vi "vPage_9222x1_CHx1.vi"() -> ()   [LabVIEW 2022 SP3]
uses:
  <vilib>/Utility/sysdir.llb/System Directory Type.ctl
  <vilib>/express/express analysis/Spectral/Block/exnSpectralBlock spectral measurements peak poly.vi
  <vilib>/express/express analysis/Spectral/Block/exnSpectralBlock spectral measurements peak DDT.vi
  <vilib>/express/express analysis/Spectral/XNode/ExpressSpectralMeasurementsBlockNode.xnode
panel:
  out "Buffer":i32
  in  "device name":tag="cDAQ8Mod1"
  in  "FFT":bool
  in  "¸ê®Æ§¨\nµù°O>":string
  out "DAQ Stoped":bool
  in  "Sample \nto Read":i32=200000
  in  "Sample\nRate":dbl=200000.0
  in  "Enable Saving":bool
  in  "Stop":bool
  out "C1-Save":bool
  out "C1-Trigger":bool
  out "C1-0":dynamicdata(graph)
  out "C1-1":dynamicdata(graph)
  # "關閉FFT\n可提高效率"
  # "當 Buffer 不為零時\n存檔&畫面會有延遲"
  # "本頁畫面顯示為 觸發後訊號"
  # "FFT Filter by useing High-pass with Lower Cut-Off (Hz)"
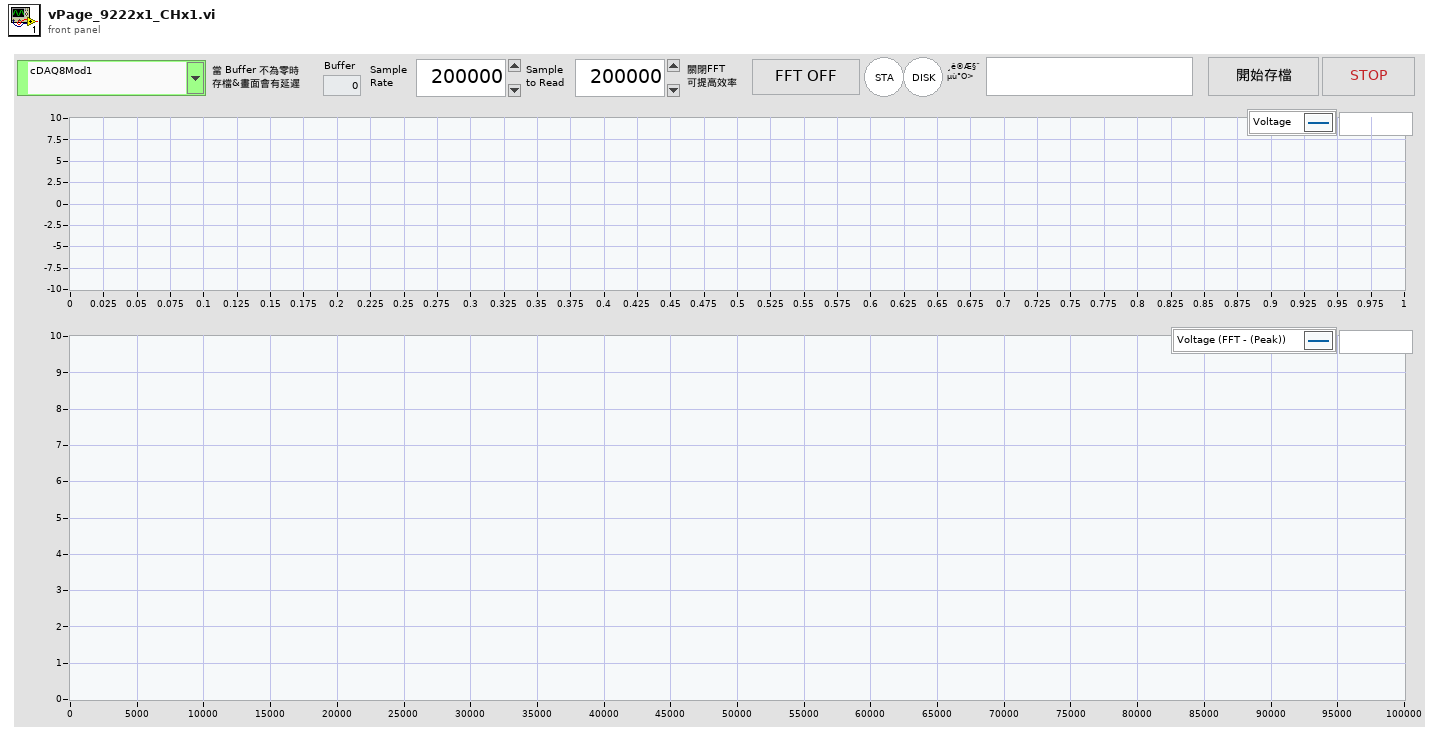
[diagram p1: front panel]
types:
  T1 = enum8{"Enabled", "Disabled", "Disabled and Grayed Out"}
  T2 = typedef "System Directory Type.ctl" = i32
  T3 = cluster{"task out":refnum<k21>, "data":dynamicdata}
  T4 = cluster{"averaging mode":u16, "weighting mode":u16, "number of averages":u32}
  T5 = cluster{"dB On (F)":bool, "unwrap phase (F)":bool, "convert to degree (F)":bool}
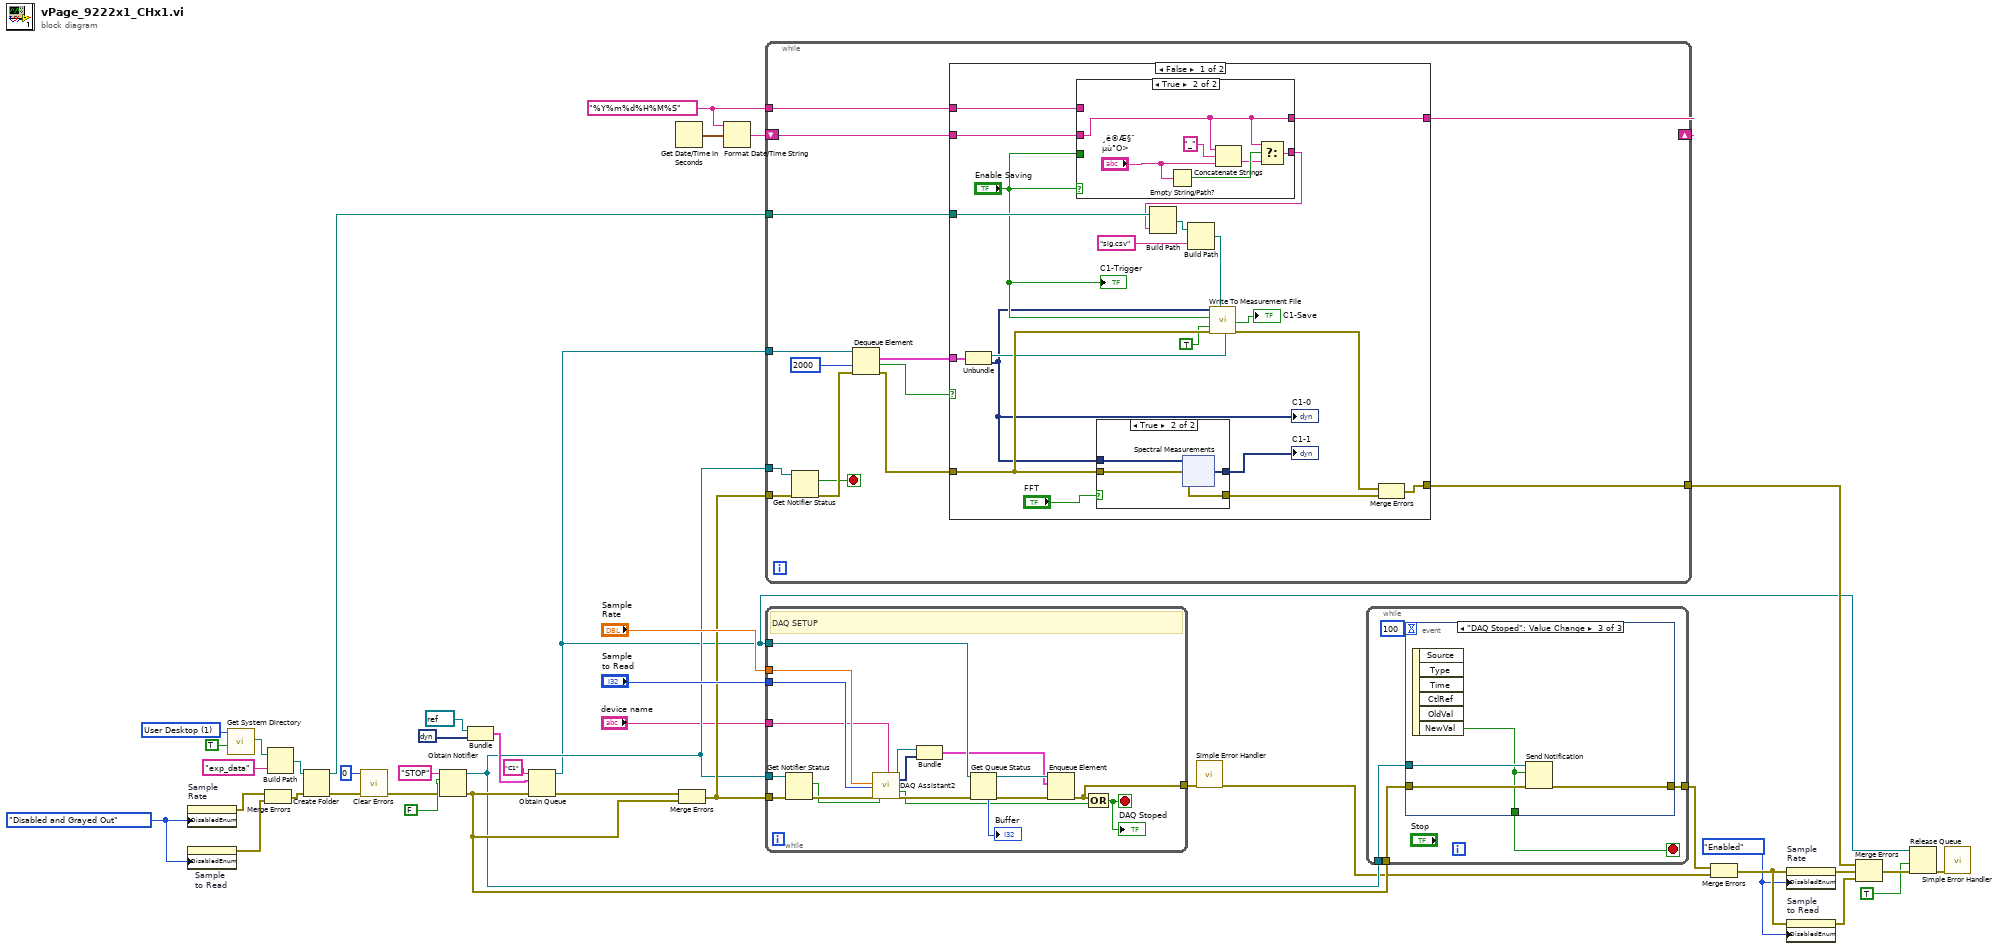
[diagram p0: block diagram]
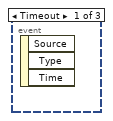
[diagram p2: hidden frame]
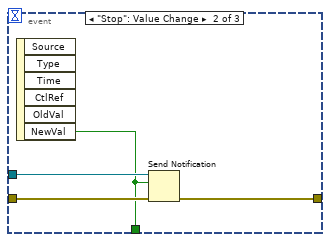
[diagram p3: hidden frame]
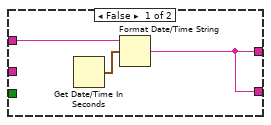
[diagram p5: hidden frame]
diagram:
  w11 = T1."Enabled" ("Disabled")
  w16 = T1."Disabled and Grayed Out" ("Disabled")
  w17 = "%Y%m%d%H%M%S" ("time format string (%c)")
  w26 = T2 1 items=["User Home"=0, "User Desktop"=1, "User Documents"=2, "User Application Data"=3, "User Preferences"=4, "User Temporary"=5, "Public Documents"=6, "Public Application Data"=7, "Public Preferences"=8, "Public Cache"=13, "System Core Libraries"=9, "System Installed Libraries"=10, "Application Files"=11, "Boot Volume Root"=12] ("system directory type")
  n1 = property on="Sample\nRate" class="DigNum (strict)"("DisabledEnum"=w16) -> (error out=w15:errorcluster)  [unwired: 2 in, 1 out]
  n2 = property on="Sample \nto Read" class="DigNum (strict)"("DisabledEnum"=w16) -> (error out=w13:errorcluster)  [unwired: 2 in, 1 out]
  n3 = call <vilib>:"Get System Directory.vi"("create directory if not found? (F)"=TRUE, "system directory type"=w26) -> ("system directory"=w28:path)  [unwired: 9 in]
  n4 = Merge Errors(w15, w13) -> (w14:errorcluster)
  n5 = Build Path(base path=w28, name or relative path="exp_data") -> (appended path=w22:path)
  n6 = Create Folder(path (use dialog)=w22, error in=w14) -> (created path=w21:path, error out=w24:errorcluster)  [unwired: 1 in, 1 out]
  n7 = call <vilib>:"Clear Errors.vi"("error in (no error)"=w24, "specific error code to clear (0: all)"=0) -> ("error out"=w23:errorcluster)  [unwired: 4 in, 1 out]
  n8 = Obtain Notifier(name (unnamed)="STOP", notification data type=FALSE, error in (no error)=w23) -> (notifier out=w18:refnum<notifier>, error out=w20:errorcluster)  [unwired: 1 in, 1 out]
  n9 = Bundle("task out"=refnum<k21> refnum, "data"=dynamicdata []) -> (w33:T3)  [unwired: 1 in]
  n10 = Obtain Queue(name (unnamed)="C1", element data type=w33, error in (no error)=w20) -> (queue out=w5:refnum<queue>, error out=w41:errorcluster)  [unwired: 2 in, 1 out]
  n11 = Get Date/Time In Seconds() -> (seconds since 1Jan1904=w31:timestamp)
  n12 = Merge Errors(w41, w20) -> (w32:errorcluster)
  n13 = Format Date/Time String(time format string (%c)=w17, seconds (now)=w31) -> (date/time string=w30:string)  [unwired: 1 in]
  n14 = while {
    tunnel: w32 -> [w55]
    tunnel: w18 -> [w53]
    tunnel: w5 -> [w52]
    shift-right: [w42] -> _
    shift-left: w30 -> [w46]
    tunnel: w21 -> [w47]
    tunnel: [w43] -> w6
    tunnel: w17 -> [w45]
    stop <- w50 stop-if-true
    n15 = Get Notifier Status(notifier=w53, error in (no error)=w55) -> (current notification=w50:bool, error out=w54:errorcluster)  [unwired: 3 out]
    n16 = Dequeue Element(queue=w52, timeout in ms (-1)=2000, error in (no error)=w54) -> (element=w48:T3, timed out?=w49:bool, error out=w44:errorcluster)  [unwired: 1 out]
    n17 = case shown="False" w49 {
      tunnel: w48 -> [w75 _]
      tunnel: w44 -> [w74 w100]
      tunnel: w46 -> [w72 w101]
      tunnel: [w71 w101] -> w42
      tunnel: w47 -> [w70 _]
      tunnel: [w64 w100] -> w43
      tunnel: w45 -> [w62 _]
      frame False {
        n18 = Unbundle(w75) -> ("task out"=w73:refnum<k21>, "data"=w60:dynamicdata)
        "C1-0" <- w60
        n19 = case shown="True" "Enable Saving" {
          tunnel: [w91 w95] -> w71
          tunnel: "Enable Saving" -> [_ _]
          tunnel: w72 -> [_ w95]
          tunnel: [w91 w97] -> w63
          tunnel: w62 -> [w92 _]
          frame False {
            n20 = Get Date/Time In Seconds() -> (seconds since 1Jan1904=w93:timestamp)
            n21 = Format Date/Time String(time format string (%c)=w92, seconds (now)=w93) -> (date/time string=w91:string)  [unwired: 1 in]
          }
          frame True {
            n22 = Empty String/Path?(string/path="¸ê®Æ§¨\nµù°O>") -> (empty?=w99:bool)
            n23 = Concatenate Strings(w95, "_" ("string"), "¸ê®Æ§¨\nµù°O>") -> (w98:string)
            n24 = Select(t=w95, s=w99, f=w98) -> (s? t:f=w97:string)
          }
        }
        n25 = case shown="True" "FFT" {
          tunnel: w74 -> [w76 w80]
          tunnel: [w76 w79] -> w65
          tunnel: [_ w78] -> w59
          tunnel: w60 -> [_ w77]
          frame False {
          }
          frame True {
            n26 = xnode ("Spectral Measurements")("Signals"=w77, "error in (no error)"=w80) -> ("FFT - (Peak)"=w78:dynamicdata, "error out"=w79:errorcluster)  [unwired: 1 out]
          }
        }
        "C1-1" <- w59
        n27 = Build Path(base path=w70, name or relative path=w63) -> (appended path=w69:path)
        n28 = Build Path(base path=w69, name or relative path="sig.csv") -> (appended path=w67:path)
        n29 = call "Write To Measurement File"("Signals"=w60, "Enable"="Enable Saving", "new_file"=TRUE, "error in (no error)"=w74, "Filename"=w67, "DAQmx Task"=w73) -> ("Saving Data"=→"C1-Save":bool, "error out"=w66:errorcluster)  [unwired: 11 in, 1 out]
        n30 = Merge Errors(w66, w65) -> (w64:errorcluster)
        "C1-Trigger" <- "Enable Saving"
      }
      frame True {
      }
    }
  }
  n31 = while {
    tunnel: [w118] -> w2
    tunnel: w5 -> [w115]
    tunnel: w32 -> [w114]
    tunnel: w18 -> [w113]
    tunnel: "Sample \nto Read" -> [w107]
    tunnel: "Sample\nRate" -> [w108]
    tunnel: "device name" -> [w102]
    stop <- w116 stop-if-true
    # "DAQ SETUP"
    n32 = Get Notifier Status(notifier=w113, error in (no error)=w114) -> (current notification=w106:bool, error out=w110:errorcluster)  [unwired: 3 out]
    n33 = call "DAQ Assistant2"("rate"=w108, "number of samples"=w107, "error in"=w110, "stop (F)"=w106, "device name"=w102) -> ("task out"=w104:refnum<k21>, "data"=w103:dynamicdata, "stopped"=w105:bool, "error out"=w109:errorcluster)  [unwired: 11 in]
    n34 = Bundle("task out"=w104, "data"=w103) -> (w111:T3)  [unwired: 1 in]
    n35 = Get Queue Status(queue=w115, error in (no error)=w109) -> (queue out=w112:refnum<queue>, error out=w119:errorcluster, # elements in queue=→"Buffer":i32)  [unwired: 1 in, 5 out]
    n36 = Enqueue Element(queue=w112, element=w111, error in (no error)=w119) -> (error out=w118:errorcluster)  [unwired: 1 in, 2 out]
    n37 = Compound Arithmetic op=OR(w118, w105) -> (w116:bool)
    "DAQ Stoped" <- w116
  }
  n38 = call <vilib>:"Simple Error Handler.vi"("error in (no error)"=w2) -> ("error out"=w1:errorcluster)  [unwired: 4 in, 4 out]
  n39 = while {
    tunnel: w20 -> [w124]
    tunnel: [w123] -> w19
    tunnel: w18 -> [w122]
    stop <- w121 stop-if-true
    n40 = event shown="[2] \"DAQ Stoped\": Value Change" {
      selector: _ -> [_ _ _]
      dyn-events: _ -> [_ _ _]
      timeout: 100 -> [_ _ _]
      tunnel: w124 -> [_ w128 w132]
      tunnel: [_ w127 w131] -> w123
      tunnel: w122 -> [_ w126 w130]
      tunnel: [_ w125 w129] -> w121
      event Timeout {
        n41 = event-data() -> ()  [unwired: 1 in, 3 out]
      }
      event "Stop": Value Change {
        n42 = event-data() -> ("NewVal"=w125:bool)  [unwired: 1 in, 5 out]
        n43 = Send Notification(notification=w125, notifier=w126, error in (no error)=w128) -> (error out=w127:errorcluster)  [unwired: 1 out]
      }
      event "DAQ Stoped": Value Change {
        n44 = event-data() -> ("NewVal"=w129:bool)  [unwired: 1 in, 5 out]
        n45 = Send Notification(notification=w129, notifier=w130, error in (no error)=w132) -> (error out=w131:errorcluster)  [unwired: 1 out]
      }
    }
  }
  n46 = Merge Errors(w19, w1) -> (w12:errorcluster)
  n47 = property on="Sample\nRate" class="DigNum (strict)"(error in=w12, "DisabledEnum"=w11) -> (error out=w10:errorcluster)  [unwired: 1 in, 1 out]
  n48 = property on="Sample \nto Read" class="DigNum (strict)"(error in=w12, "DisabledEnum"=w11) -> (error out=w9:errorcluster)  [unwired: 1 in, 1 out]
  n49 = Merge Errors(w6, w10, w9) -> (w7:errorcluster)
  n50 = Release Queue(queue=w5, force destroy? (F)=TRUE, error in (no error)=w7) -> (error out=w8:errorcluster)  [unwired: 2 out]
  n51 = call <vilib>:"Simple Error Handler.vi"("error in (no error)"=w8) -> ()  [unwired: 4 in, 5 out]
